vi "Hardware-IRQControlCalPoints.vi"() -> (3 "IRQs":T1[](array[typedef]))   [LabVIEW 2016, in "DSI-RT.lvlib"]
uses:
  DSI-RT.lvlib
  <vilib>/Powertrain Controls/Device Drivers/DCM/IRQ/RT/IRQ Setup.ctl
  <vilib>/addons/Software Calibration Management/xSCM/CalPoint.xnode
  <vilib>/addons/Software Calibration Management/xSCM/ni_scm.dll
  <vilib>/Powertrain Controls/Device Drivers/DCM/IRQ/RT/DCM - RT - IRQ.lvlib
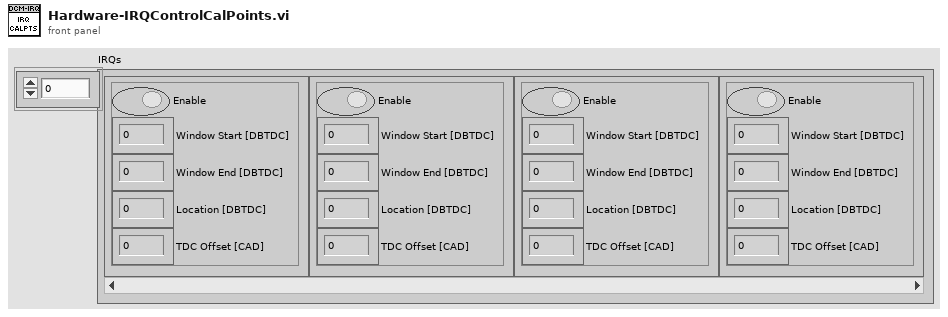
[diagram p1: front panel]
types:
  T1 = typedef "DCM - RT - IRQ.lvlib/IRQ Setup.ctl" = cluster{"Enable":bool, "Window Start [DBTDC]":sgl, "Window End [DBTDC]":sgl, "Location [DBTDC]":sgl, "TDC Offset [CAD]":sgl}
  T2 = cluster{"Enable":bool, "Window Start [DBTDC]":sgl, "Window End [DBTDC]":sgl, "Location [DBTDC]":sgl, "TDC Offset [CAD]":sgl}[]
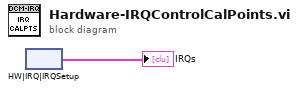
[diagram p0: block diagram]
diagram:
  n1 = xnode "HW|IRQ|IRQSetup"() -> ("Value"=→"IRQs":T2)
